vi "SV TDMS Read Waveform (1 Ch).vi"(0 "tdms file":refnum<k34>, 1 "offset (0)":i64, 2 "count (-1: all)":i64=-1, 5 "group name in":string, 7 "channel name in":string, 11 "error in":errorcluster) -> (4 "tdms file out":refnum<k34>, 6 "group name out":string, 8 "channel name out":string, 10 "waveform":waveform(dbl), 14 "eof":bool, 15 "error out":errorcluster)   [LabVIEW 2017]
doc: "Reads the specified .tdms file and returns data in a format specific to the polymorphic instance selected."
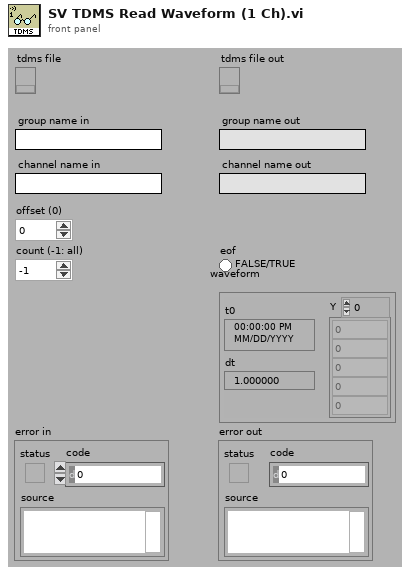
[diagram p1: front panel]
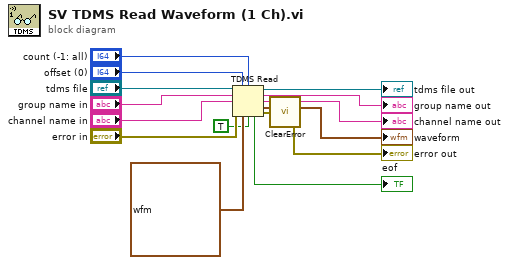
[diagram p0: block diagram]
diagram:
  n1 = TDMS Read(0:"tdms file", 1:"offset (0)", 2:"count (-1: all)", 5:"group name in", 7:"channel name in", 11:"error in", 12:waveform(dbl) {"t0"=timestamp(-18000 s since 1904-01-01), "dt"=1.0, "Y"=[]} ("waveform"), 13:TRUE ("return channels in file order? (F)")) -> (4:→"tdms file out":refnum<k34>, 6:→"group name out":string, 8:→"channel name out":string, 10:→"waveform":waveform(dbl), 14:→"eof":bool, 15:w2:errorcluster)
  n2 = call <vilib>:"ClearError.vi"("error in (no error)"=w2) -> ("error out"=→"error out":errorcluster)
